vi "Shoot Ball.vi"(9 "SolenoidDevRef":T1={"DevStatus"={"status"=FALSE, "code"=0, "source"=""}, "Pneumatics Control Module"=0, "Forward Solenoid Channel"=enum."Invalid", "Reverse Solenoid Channel"=enum."Invalid"}, 11 "Iteration":i32) -> (1 "Speed":dbl, 3 "Finished":bool)   [LabVIEW 2016]
uses:
  <vilib>/Rock Robotics/WPI/Solenoid/WPI_SolenoidDevRef.ctl
  <vilib>/Rock Robotics/WPI/Solenoid/WPI_SolenoidChannel.ctl
  <vilib>/Rock Robotics/WPI/Solenoid/WPI_SolenoidValue.ctl
  <vilib>/Rock Robotics/WPI/Solenoid/WPI_SolenoidSetEnum.vi
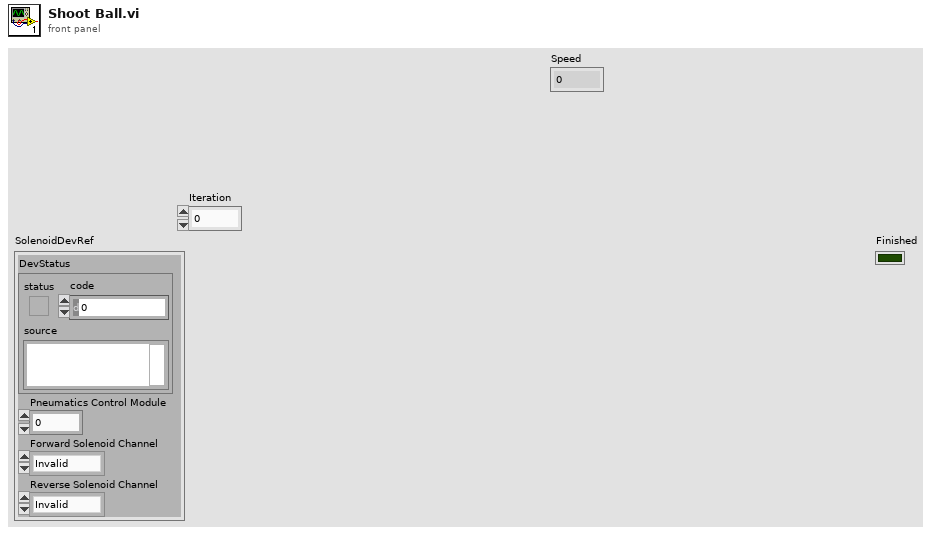
[diagram p1: front panel]
types:
  T1 = typedef "WPI_SolenoidDevRef.ctl" = cluster{"DevStatus":errorcluster, "Pneumatics Control Module":u8, "Forward Solenoid Channel":T2, "Reverse Solenoid Channel":T2}
  T2 = typedef "WPI_SolenoidChannel.ctl" = enum8{"Solenoid 0", "Solenoid 1", "Solenoid 2", "Solenoid 3", "Solenoid 4", "Solenoid 5", "Solenoid 6", "Solenoid 7", "Invalid"}
  T3 = typedef "WPI_SolenoidValue.ctl" = enum16{"Off", "On", "Forward", "Reverse"}
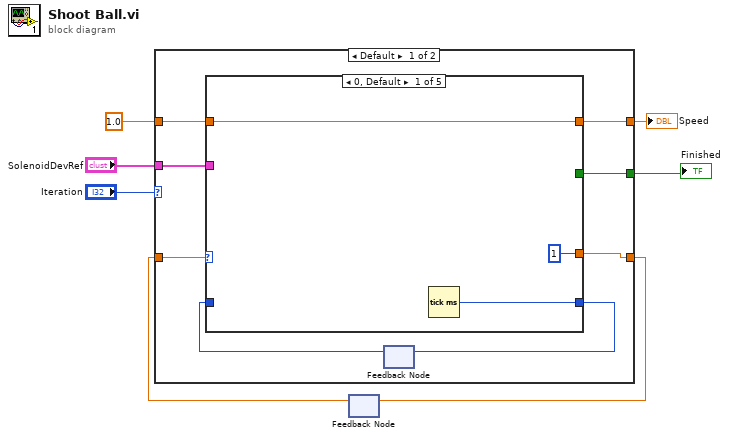
[diagram p0: block diagram]
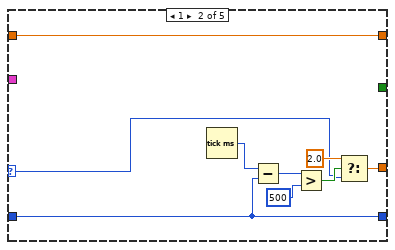
[diagram p2: hidden frame]
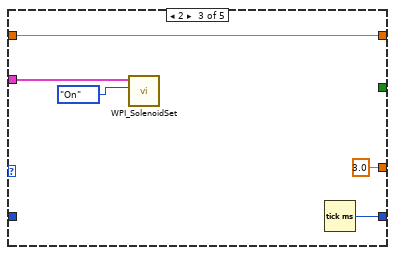
[diagram p3: hidden frame]
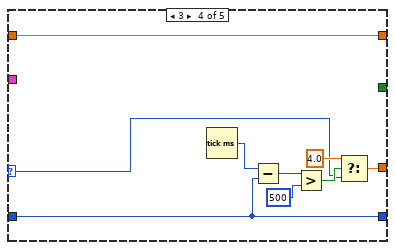
[diagram p4: hidden frame]
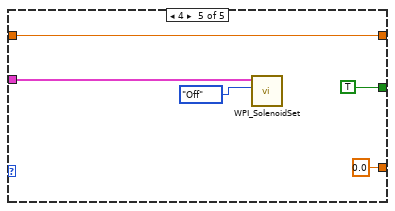
[diagram p5: hidden frame]
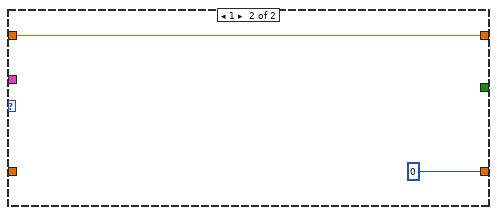
[diagram p6: hidden frame]
diagram:
  n1 = feedback #1() -> (w5:dbl)  [unwired: 1 in]
  n2 = case shown="Default" "Iteration" {
    tunnel: [w10 0] -> w6
    tunnel: w5 -> [w15 _]
    tunnel: 1.0 -> [w14 w47]
    tunnel: [w13 w47] -> w3
    tunnel: "SolenoidDevRef" -> [w9 _]
    tunnel: [w8 _] -> w1
    frame Default {
      n3 = feedback #2() -> (w11:u32)  [unwired: 1 in]
      n4 = case shown="0, Default" w15 {
        selector: w15 -> [_ w20 _ w34 _]
        tunnel: w14 -> [w16 w19 w29 w33 w43]
        tunnel: [w16 w19 w29 w33 w43] -> w13
        tunnel: [w18 w26 w30 w40 _] -> w12
        tunnel: w11 -> [_ w26 _ w40 _]
        tunnel: [1 w23 3.0 ("t") w37 0.0 ("t")] -> w10
        tunnel: w9 -> [_ _ w32 _ w44]
        tunnel: [_ _ _ _ TRUE] -> w8
        frame 0, Default {
          n5 = Tick Count (ms)() -> (millisecond timer value=w18:u32)
        }
        frame 1 {
          n6 = Tick Count (ms)() -> (millisecond timer value=w27:u32)
          n7 = Subtract(x=w27, y=w26) -> (x-y=w25:u32)
          n8 = Greater?(x=w25, y=u32 500) -> (0:w21:bool)
          n9 = Select(t=2.0, s=w21, f=w20) -> (s? t:f=w23:dbl)
        }
        frame 2 {
          n10 = call-poly <vilib>:"WPI_SolenoidSet.vi"("Value"=WPI_SolenoidValue."On", "SolenoidDevRef"=w32) -> ()  [unwired: 8 in, 2 out]
          n11 = Tick Count (ms)() -> (millisecond timer value=w30:u32)
        }
        frame 3 {
          n12 = Tick Count (ms)() -> (millisecond timer value=w41:u32)
          n13 = Subtract(x=w41, y=w40) -> (x-y=w39:u32)
          n14 = Greater?(x=w39, y=u32 500) -> (0:w35:bool)
          n15 = Select(t=4.0, s=w35, f=w34) -> (s? t:f=w37:dbl)
        }
        frame 4 {
          n16 = call-poly <vilib>:"WPI_SolenoidSet.vi"("Value"=WPI_SolenoidValue."Off", "SolenoidDevRef"=w44) -> ()  [unwired: 8 in, 2 out]
        }
      }
      n17 = feedback-in #2(w12) -> ()
    }
    frame 1 {
    }
  }
  "Speed" <- w3
  "Finished" <- w1
  n18 = feedback-in #1(w6) -> ()
